vi "AcPwrState.vi"(7 "Set":bool, 11 "strngStateIn":string caption="State In") -> (3 "strngStateOut":string caption="State Out")   [LabVIEW 2014, in "AcPwrModule.lvlib"]
uses:
  AcPwrModule.lvlib
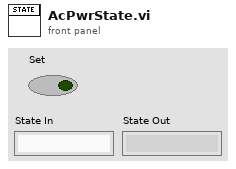
[diagram p1: front panel]
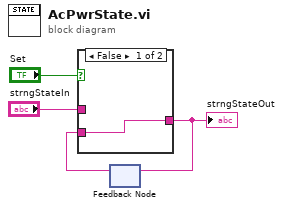
[diagram p0: block diagram]
diagram:
  n1 = feedback #1() -> (w1:string)  [unwired: 1 in]
  n2 = case shown="False" "Set" {
    tunnel: [w5 w6] -> w2
    tunnel: "strngStateIn" -> [_ w6]
    tunnel: w1 -> [w5 _]
    frame False {
    }
    frame True {
    }
  }
  "strngStateOut" <- w2
  n3 = feedback-in #1(w2) -> ()
